vi "Shooter Testing.vi"() -> ()   [LabVIEW 2012]
panel:
  in  "Shooter Test Speed":dbl
  in  "Shooter Test?":bool
  # "Use button 12 to test the shooter. For shooter test speed to work,\nyou have to enable the 'shooter test' boolean."
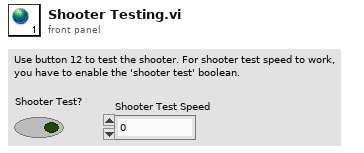
[diagram p1: front panel]
diagram:
